vi "PicoScope9400_Test_Get_Data.vi"(11 "ExecCommand":string="WFM:SOURCE CH1;DATA -0.041675, -0.002425, -0.19755, -0.0363, -0.1523, 0.022325, 0.098325, 0.073325, 0.11457, -0.0863, 0.05995, -0.071175, -0.019425, 0.052575, 0.11083, 0.057325, 0.003825, 0.009325, 0.077075, 0.002575, -0.091425, 0.094075, -0.085675, 0.0472, -0.0003, -0.053925, -0.0723, -0.03655, 0.1722, -0.11155, -0.013925, 0.041575, 0.062825, -0.012675, -0.0073, -0.0038, -0.1028, -0.0043, -0.020175, 0.005825, 0.05395, 0.10245, 0.11145, 0.0172, 0.058575, -0.01755, 0.16595, 0.13645, 0.023075, 0.019825, 0.007575, 0.10258, 0.1157, -0.042425, -0.055425, 0.0387, 0.056575, -0.02155, 0.049825, 0.083575, 0.12495, -0.086675, 0.001325, -0.035175, -0.1738, 0.05995, 0.10783, -0.15143, 0.16833, -0.0223, 0.018075, -0.086425, -0.12755, -0.10855, -0.15018, -0.019175, 0.0097, 0.00695, -0.1563, -0.076925, 0.04195, -0.04305, 0.04745, -0.1228, -0.02155, -0.03705, -0.05305, 0.051575, 0.13695, 0.013825, -0.047425, 0.003825, -0.0183, 0.072325, 0.0257, -0.03805, -0.055675, 0.070825, -0.0853, -0.09105, -0.052925, -0.0143, 0.052575, -0.11755, -0.015675, 0.06445, -0.1058, 0.08345, -0.11217, 0.09095, -0.12205, 0.0097, 0.039825, -0.056425, 0.12395, -0.0108, 0.0277, 0.15695, 0.0572, 0.0747, -0.013675, -0.05605, 0.017325, 0.0547, 0.022075, -0.01505, -0.006675, 0.04795, 0.14208, -0.064175, -0.037925, 0.0622, 0.025325, -0.008925, -0.013925, 0.00445, 0.012075, -0.10105, -0.07655, -0.0218, 0.0597, 0.0997, -0.002925, 0.10945, -0.075425, -0.024675, -0.06105, 0.094325, 0.020575, 0.044575, -0.0773, 0.021075, -0.11105, -0.06505, -0.0383, -0.11718, -0.0088, -0.083925, -0.09105, 0.00445, -0.05405, 0.064825, 0.06145, 0.14183, 0.07945, -0.02855, -0.02255, -0.026175, 0.0302, -0.0143, -0.11292, -0.060675, -0.070925, -0.0718, -0.099425, 0.0077, -0.045925, 0.020075, -0.13517, -0.0743, -0.10818, 0.003075, 0.01795, -0.1138, -0.043925, -0.04855, -0.003925, 0.018825, -0.055675, 0.1022, -0.13118, 0.14695, 0.03245, -0.092675, -0.0338, -0.0943, -0.00355, -0.13355, 0.010825, 0.001575, 0.13545, -0.01905, -0.12743, -0.01155, -0.019675, 0.080575, 0.11545, -0.034925, 0.06395, 0.19045, 0.054075, 0.15957, 0.080575, -0.1103, -0.04605, -0.09855, -0.14167, -0.0208, 0.027325, 0.002825, 0.002075, 0.0977, -0.0218, -0.0478, 0.007825, 0.01645, 0.10933, 0.056575, 0.0112, -0.008175, -0.029675, 0.0172, 0.11395, -0.05105, 0.057575, -0.0658, 0.002325, -0.03105, -0.0033, -0.076175, -0.07555, -0.0108, -0.015175, 0.027075, -0.00255, -0.2078, -0.01205, -0.07155, -0.0088, -0.10293, -0.0438, 0.035575, -0.07355, -0.17918, -0.06555, -0.034425, -0.017675, -0.0908, -0.04855, -0.0058, -0.052175, 0.1027, 0.053825, -0.0098, 0.0807, 0.0547, -0.082675, -0.026175, -0.0618, 0.087825, -0.02905, -0.05405, 0.15283, -0.0043, 0.09595, -0.075675, -0.0758, 0.04595, 0.20758, 0.047575, 0.03145, -0.024675, 0.0027, 0.066575, 0.0307, 0.0642, -0.01755, -0.0858, -0.0843, -0.05205, 0.094575, -0.0648, -0.046175, -0.012175, -0.072425, -0.057925, 0.084325, -0.078425, 0.0547, 0.082575, 0.006325, 0.02295, 0.11383, 0.087075, 0.035325, 0.01695, -0.0623, -0.075425, 0.02745, -0.0193, -0.00505, 0.086075, 0.08645, 0.03745, 0.086575, 0.07295, 0.046825, 0.11133, 0.0212, -0.024925, -0.05355, -0.0238, -0.0548, 0.13057, 0.12433, -0.12793, 0.0992, -0.0883, 0.11995, -0.0353, -0.0258, -0.005925, 0.0302, 0.13207, -0.0113, 0.076075, -0.05355, 0.10733, 0.11995, -0.02055, -0.009175, 0.01045, -0.048675, 0.0407, -0.0158, -0.001925, -0.0503, 0.0962, -0.030925, 0.11345, -0.019425, -0.12005, 0.0747, 0.0547, 0.15895, 0.34508, 0.37057, 0.4687, 0.52182, 0.4652, 0.6007, 0.59545, 0.4587, 0.40445, 0.3862, 0.37857, 0.4332, 0.50895, 0.4117, 0.53107, 0.47883, 0.42933, 0.4917, 0.49895, 0.5702, 0.60433, 0.5062, 0.36395, 0.46682, 0.4137, 0.5887, 0.57595, 0.59532, 0.47658, 0.5367, 0.61483, 0.52382, 0.6142, 0.4582, 0.5267, 0.54045, 0.45695, 0.39033, 0.52195, 0.42945, 0.6172, 0.66007, 0.51782, 0.5132, 0.4842, 0.50657, 0.57483, 0.46082, 0.43895, 0.13933, 0.086325, 0.076075, 0.12557, -0.06355, 0.0972, 0.057325, 0.0767, -0.036175, 0.03095, -0.10668, 0.01045, -0.0443, -0.0168, -0.071675, -0.013675, -0.097675, -0.0383, -0.1608, 0.053075, -0.00155, 0.10157, -0.10305, 0.079825, 0.05345, 0.089325, 0.064575, -0.05555, -0.0153, -0.045675, -0.003925, 0.14358, -0.12443, -0.09155, -0.063175, 0.066325, -0.076425, 0.025825, 0.0612, -0.02305, 0.03945, -0.077675, -0.038675, 0.11795, -0.08905, 0.030575, -0.0368, -0.042925, 0.027575, 0.003075, -0.08655, 0.0597, -0.00105, 0.074325, 0.24733, 0.010825, 0.013325, 0.055075, -0.0158, 0.02745, -0.03905, 0.0342, -0.054425, 0.08445, 0.008575, 0.1772, -0.00505, -0.12743, -0.10355, -0.12243, 0.0072, -0.043925, -0.097425, 0.07695, 0.07245, -0.03455, -0.0573, 0.1062, 0.0077, 0.06895, -0.02255, -0.1003, 0.092325, 0.24345, 0.022325, 0.10308, -0.038675, 0.035075, 0.010825, 0.0327, 0.01245, -0.12855, 0.10645, 0.051825, -0.0048, -0.03105, 0.018075, 0.10995, 0.061575, -0.097675, -0.026925, 0.0182, 0.10908, -0.092425, 0.020825, -0.0113, -0.00705, 0.086325, ;\r\nPREAMB: Points = 512, XInc = 2E-11, XOrig = 0, XU = s, YU = V;\r\nCOMPLEX MOD") -> (0 "XU":string, 1 "Data Array":sgl[](array[numeric]), 2 "Xint":sgl format="%_6e", 3 "Xmin":sgl format="%_6e", 4 "Ymin":sgl, 5 "Xmax":sgl, 6 "Ymax":sgl, 7 "Data":string, 8 "YU":string)   [LabVIEW 2013]
panel:
  out "Point":sgl
  out "YU":string
  out "XU":string
  out "Xorig":string
  out "Xint":string
  out "Point":string
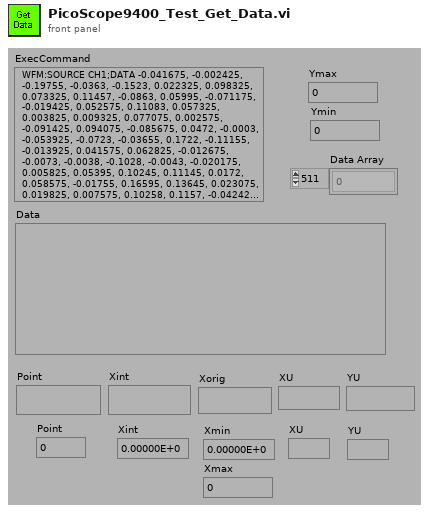
[diagram p1: front panel]
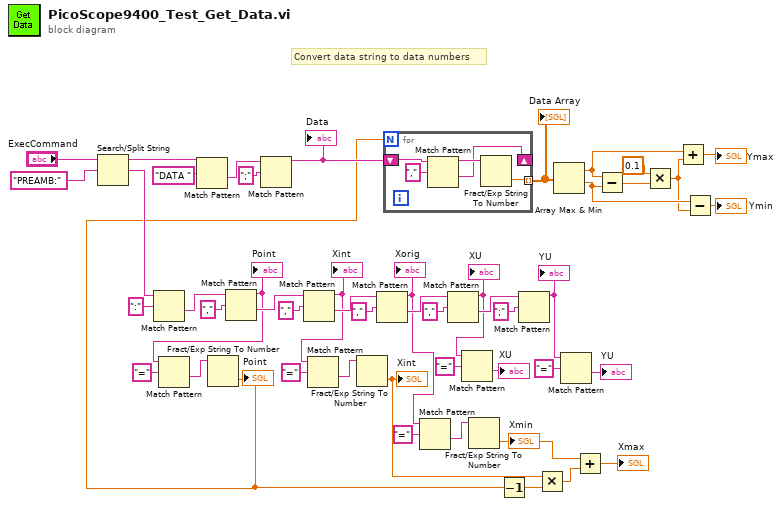
[diagram p0: block diagram]
diagram:
  # "Convert data string to data numbers"
  n1 = Search/Split String(string="ExecCommand", search string/char (-)="PREAMB:") -> (substring before match=w33:string, match + rest of string=w44:string)  [unwired: 1 in, 1 out]
  n2 = Match Pattern(string=w44, regular expression=":") -> (after substring=w43:string)  [unwired: 1 in, 3 out]
  n3 = Match Pattern(string=w33, regular expression="DATA ") -> (after substring=w31:string)  [unwired: 1 in, 3 out]
  n4 = Match Pattern(string=w43, regular expression=",") -> (before substring=w15:string, after substring=w41:string)  [unwired: 1 in, 2 out]
  "Point" <- w15
  n5 = Match Pattern(string=w15, regular expression="=") -> (after substring=w16:string)  [unwired: 1 in, 3 out]
  n6 = Fract/Exp String To Number(string=w16) -> (number=w13:dbl)  [unwired: 3 in, 1 out]
  "Point" <- w13
  n7 = Match Pattern(string=w31, regular expression=";") -> (before substring=w30:string)  [unwired: 1 in, 3 out]
  "Data" <- w30
  n8 = Match Pattern(string=w41, regular expression=",") -> (before substring=w28:string, after substring=w39:string)  [unwired: 1 in, 2 out]
  "Xint" <- w28
  n9 = Match Pattern(string=w28, regular expression="=") -> (after substring=w27:string)  [unwired: 1 in, 3 out]
  n10 = Fract/Exp String To Number(string=w27) -> (number=w12:dbl)  [unwired: 3 in, 1 out]
  "Xint" <- w12
  n11 = Match Pattern(string=w39, regular expression=",") -> (before substring=w24:string, after substring=w37:string)  [unwired: 1 in, 2 out]
  "Xorig" <- w24
  n12 = for {
    N: w13 -> [_]
    shift-right: [w51] -> _
    shift-left: w30 -> [w50]
    tunnel: [w49] -> w14 mode=indexing
    n13 = Match Pattern(string=w50, regular expression=",") -> (before substring=w52:string, after substring=w51:string)  [unwired: 1 in, 2 out]
    n14 = Fract/Exp String To Number(string=w52) -> (number=w49:dbl)  [unwired: 3 in, 1 out]
  }
  "Data Array" <- w14
  n15 = Match Pattern(string=w24, regular expression="=") -> (after substring=w25:string)  [unwired: 1 in, 3 out]
  n16 = Match Pattern(string=w37, regular expression=",") -> (before substring=w21:string, after substring=w35:string)  [unwired: 1 in, 2 out]
  "XU" <- w21
  n17 = Match Pattern(string=w21, regular expression="=") -> (after substring=→"XU":string)  [unwired: 1 in, 3 out]
  n18 = Fract/Exp String To Number(string=w25) -> (number=w10:dbl)  [unwired: 3 in, 1 out]
  "Xmin" <- w10
  n19 = Decrement(x=w13) -> (x-1=w11:dbl)
  n20 = Match Pattern(string=w35, regular expression=";") -> (before substring=w19:string)  [unwired: 1 in, 3 out]
  "YU" <- w19
  n21 = Multiply(x=w12, y=w11) -> (x*y=w9:dbl)
  n22 = Array Max & Min(array=w14) -> (max value=w7:dbl, min value=w5:dbl)  [unwired: 2 out]
  n23 = Match Pattern(string=w19, regular expression="=") -> (after substring=→"YU":string)  [unwired: 1 in, 3 out]
  n24 = Add(x=w10, y=w9) -> (x+y=→"Xmax":dbl)
  n25 = Subtract(x=w7, y=w5) -> (x-y=w4:dbl)
  n26 = Multiply(x=0.1, y=w4) -> (x*y=w1:dbl)
  n27 = Add(x=w7, y=w1) -> (x+y=→"Ymax":dbl)
  n28 = Subtract(x=w5, y=w1) -> (x-y=→"Ymin":dbl)
